vi "AutoInit.vi"   [LabVIEW 2023]
doc: "Sets all robot commands to their proper intial state."
uses:
  GlobalDriverStationCommands.vi
  GlobalAutonomous.vi
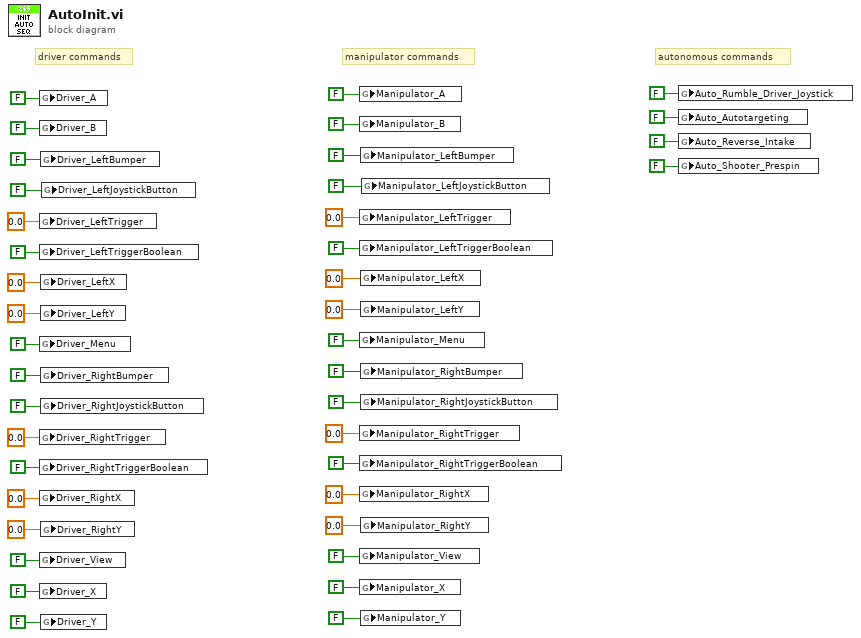
[diagram p0: block diagram]
diagram:
  # "manipulator commands"
  # "driver commands"
  # "autonomous commands"
  n1 = global write "GlobalDriverStationCommands.vi" "Driver_A"(FALSE ("Driver_A")) -> ()
  n2 = global write "GlobalDriverStationCommands.vi" "Driver_B"(FALSE ("Driver_B")) -> ()
  n3 = global write "GlobalDriverStationCommands.vi" "Driver_LeftTrigger"(0.0 ("Driver_LeftTrigger")) -> ()
  n4 = global write "GlobalDriverStationCommands.vi" "Driver_LeftTriggerBoolean"(FALSE ("Driver_LeftTriggerBoolean")) -> ()
  n5 = global write "GlobalDriverStationCommands.vi" "Driver_Menu"(FALSE ("Driver_Menu")) -> ()
  n6 = global write "GlobalDriverStationCommands.vi" "Driver_RightTrigger"(0.0 ("Driver_RightTrigger")) -> ()
  n7 = global write "GlobalDriverStationCommands.vi" "Driver_RightTriggerBoolean"(FALSE ("Driver_RightTriggerBoolean")) -> ()
  n8 = global write "GlobalDriverStationCommands.vi" "Driver_RightX"(0.0 ("Driver_RightX")) -> ()
  n9 = global write "GlobalDriverStationCommands.vi" "Driver_View"(FALSE ("Driver_View")) -> ()
  n10 = global write "GlobalDriverStationCommands.vi" "Driver_X"(FALSE ("Driver_X")) -> ()
  n11 = global write "GlobalDriverStationCommands.vi" "Driver_LeftBumper"(FALSE ("Driver_LeftBumper")) -> ()
  n12 = global write "GlobalDriverStationCommands.vi" "Driver_LeftX"(0.0 ("Driver_LeftX")) -> ()
  n13 = global write "GlobalDriverStationCommands.vi" "Driver_LeftY"(0.0 ("Driver_LeftY")) -> ()
  n14 = global write "GlobalDriverStationCommands.vi" "Driver_RightBumper"(FALSE ("Driver_RightBumper")) -> ()
  n15 = global write "GlobalDriverStationCommands.vi" "Driver_RightJoystickButton"(FALSE ("Driver_RightJoystickButton")) -> ()
  n16 = global write "GlobalDriverStationCommands.vi" "Driver_RightY"(0.0 ("Driver_RightY")) -> ()
  n17 = global write "GlobalDriverStationCommands.vi" "Driver_Y"(FALSE ("Driver_Y")) -> ()
  n18 = global write "GlobalDriverStationCommands.vi" "Driver_LeftJoystickButton"(FALSE ("Driver_LeftJoystickButton")) -> ()
  n19 = global write "GlobalDriverStationCommands.vi" "Manipulator_A"(FALSE ("Driver_A")) -> ()
  n20 = global write "GlobalDriverStationCommands.vi" "Manipulator_B"(FALSE ("Driver_B")) -> ()
  n21 = global write "GlobalDriverStationCommands.vi" "Manipulator_LeftTrigger"(0.0 ("Driver_LeftTrigger")) -> ()
  n22 = global write "GlobalDriverStationCommands.vi" "Manipulator_LeftTriggerBoolean"(FALSE ("Driver_LeftTriggerBoolean")) -> ()
  n23 = global write "GlobalDriverStationCommands.vi" "Manipulator_Menu"(FALSE ("Driver_Menu")) -> ()
  n24 = global write "GlobalDriverStationCommands.vi" "Manipulator_RightTrigger"(0.0 ("Driver_RightTrigger")) -> ()
  n25 = global write "GlobalDriverStationCommands.vi" "Manipulator_RightTriggerBoolean"(FALSE ("Driver_RightTriggerBoolean")) -> ()
  n26 = global write "GlobalDriverStationCommands.vi" "Manipulator_RightX"(0.0 ("Driver_RightX")) -> ()
  n27 = global write "GlobalDriverStationCommands.vi" "Manipulator_View"(FALSE ("Driver_View")) -> ()
  n28 = global write "GlobalDriverStationCommands.vi" "Manipulator_X"(FALSE ("Driver_X")) -> ()
  n29 = global write "GlobalDriverStationCommands.vi" "Manipulator_LeftBumper"(FALSE ("Driver_LeftBumper")) -> ()
  n30 = global write "GlobalDriverStationCommands.vi" "Manipulator_LeftX"(0.0 ("Driver_LeftX")) -> ()
  n31 = global write "GlobalDriverStationCommands.vi" "Manipulator_LeftY"(0.0 ("Driver_LeftY")) -> ()
  n32 = global write "GlobalDriverStationCommands.vi" "Manipulator_RightBumper"(FALSE ("Driver_RightBumper")) -> ()
  n33 = global write "GlobalDriverStationCommands.vi" "Manipulator_RightJoystickButton"(FALSE ("Driver_RightJoystickButton")) -> ()
  n34 = global write "GlobalDriverStationCommands.vi" "Manipulator_RightY"(0.0 ("Driver_RightY")) -> ()
  n35 = global write "GlobalDriverStationCommands.vi" "Manipulator_Y"(FALSE ("Driver_Y")) -> ()
  n36 = global write "GlobalDriverStationCommands.vi" "Manipulator_LeftJoystickButton"(FALSE ("Driver_LeftJoystickButton")) -> ()
  n37 = global write "GlobalAutonomous.vi" "Auto_Rumble_Driver_Joystick"(FALSE ("Auto_Force_To_Low_Gear")) -> ()
  n38 = global write "GlobalAutonomous.vi" "Auto_Autotargeting"(FALSE ("Auto_Autotargeting")) -> ()
  n39 = global write "GlobalAutonomous.vi" "Auto_Reverse_Intake"(FALSE) -> ()
  n40 = global write "GlobalAutonomous.vi" "Auto_Shooter_Prespin"(FALSE) -> ()
